vi "Build_Array.vi"(8 "OY":dbl[][](array[numeric]), 11 "OX":dbl[](array[numeric])) -> (0 "Other":cluster{"OX":dbl[], "OY":dbl[]}[](array[cluster]), 3 "Time":cluster{timestamp[], "OY":dbl[]}[](array[cluster]))   [LabVIEW 2023, in "Graph_data_collector.lvlib" / "Graph_UI.lvlib"]
uses:
  Graph_UI.lvlib
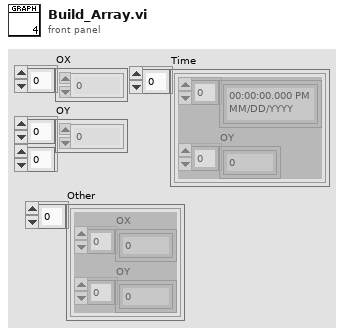
[diagram p1: front panel]
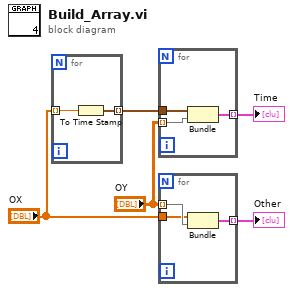
[diagram p0: block diagram]
diagram:
  n1 = for {
    tunnel: "OX" -> [w7] mode=indexing
    tunnel: [w6] -> w5 mode=indexing
    n2 = To Time Stamp(1:w7) -> (0:w6:timestamp)
  }
  n3 = for {
    tunnel: "OY" -> [w10] mode=indexing
    tunnel: [w9] -> w2 mode=indexing
    tunnel: w5 -> [w8]
    n4 = Bundle(w8, "OY"=w10) -> (w9:cluster{timestamp[], "OY":dbl[]})  [unwired: 1 in]
  }
  "Time" <- w2
  n5 = for {
    tunnel: "OY" -> [w13] mode=indexing
    tunnel: [w12] -> w1 mode=indexing
    tunnel: "OX" -> [w11]
    n6 = Bundle("OX"=w11, "OY"=w13) -> (w12:cluster{"OX":dbl[], "OY":dbl[]})  [unwired: 1 in]
  }
  "Other" <- w1
